vi "Tick.vi"(8 "error in (no error)":errorcluster, 11 "Ticker In":refnum<class "Ticker.lvclass">) -> (0 "error out":errorcluster, 3 "Ticker Out":refnum<class "Ticker.lvclass">)   [LabVIEW 2025, in "Ticker.lvclass"]
uses:
  Ticker.lvclass
  Ticker.lvclass/Ticker.ctl
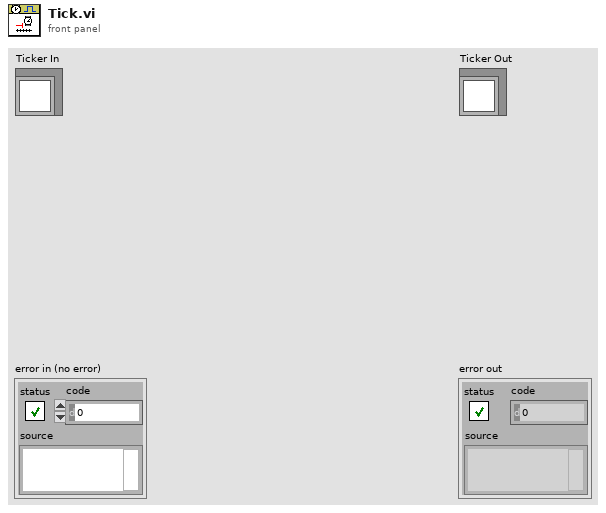
[diagram p1: front panel]
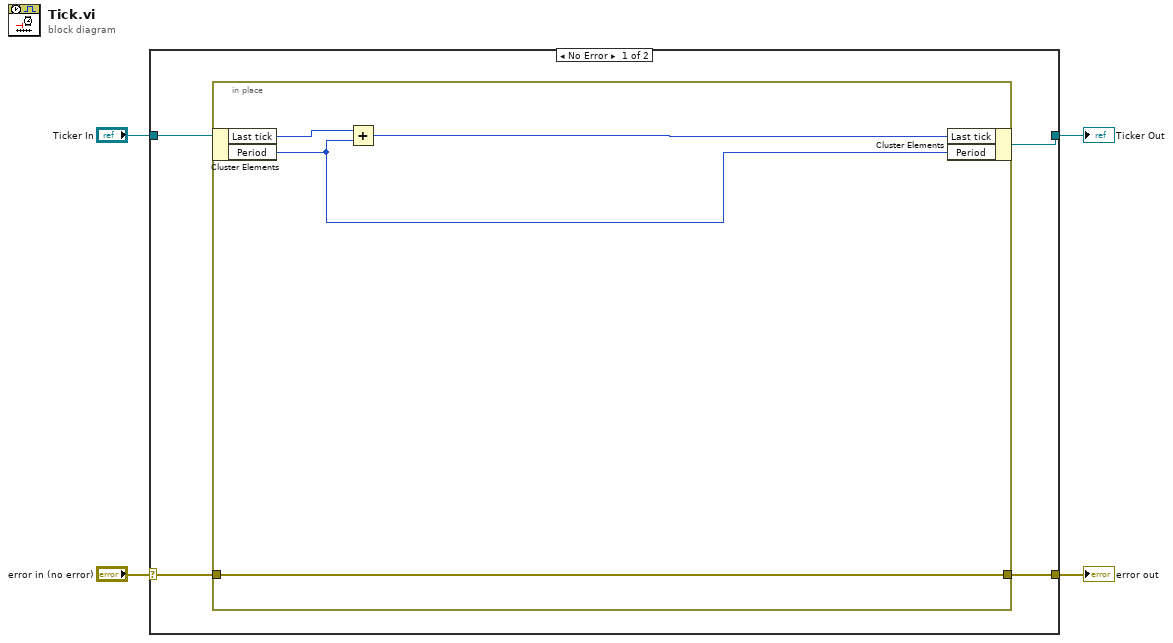
[diagram p0: block diagram]
diagram:
  n1 = case shown="No Error" "error in (no error)" {
    selector: "error in (no error)" -> [w5 w14]
    tunnel: [w6 w14] -> w2
    tunnel: [w7 w13] -> w3
    tunnel: "Ticker In" -> [w8 w13]
    frame No Error {
      n2 = in-place {
        in-place-border: [w12] -> w6
        in-place-border: w5 -> [w12]
        n3 = in-place-cluster #1(w8) -> ("Last tick"=w10:u32, "Period"=w9:u32)
        n4 = Add(x=w10, y=w9) -> (x+y=w11:u32)
        n5 = in-place-cluster #1("Last tick"=w11, "Period"=w9) -> (w7:refnum<class "Ticker.lvclass">)
      }
    }
    frame Error {
    }
  }
  "error out" <- w2
  "Ticker Out" <- w3
